vi "hse-application__GetSingleton.vi"(11 "Action":T1=enum."Get") -> (0 "Error Out":errorcluster, 3 "ApplicationClass DVR":refnum<data-value>)   [LabVIEW 2014, in "hse-application.lvclass"]
doc: "Contains the DVR to the HSE ApplicationClass object.\n\n____\nHAMPEL SOFTWARE ENGINEERING v0.12.0 (2018-09-13 18:21)"
uses:
  hse-application.lvclass
  hse-misc/Controls/FGV_Actions.ctl
  hse-misc/hse-misc.lvlib
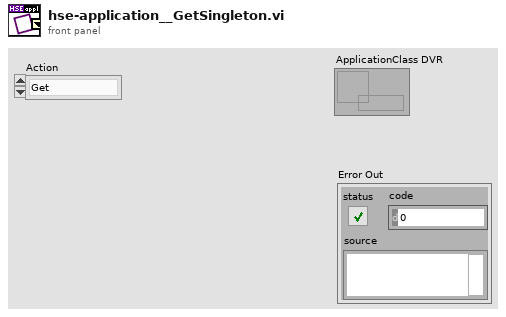
[diagram p1: front panel]
types:
  T1 = typedef "hse-misc.lvlib/FGV_Actions.ctl" = enum16{"Set", "Get"}
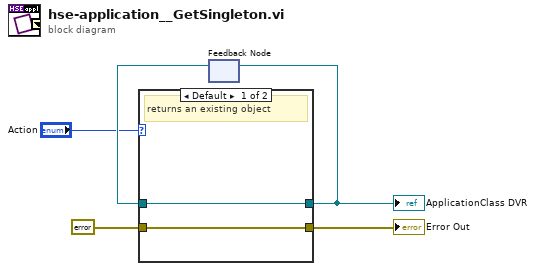
[diagram p0: block diagram]
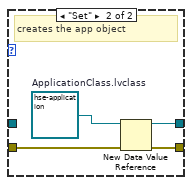
[diagram p2: hidden frame]
diagram:
  n1 = feedback #1() -> (w4:refnum<data-value>)  [unwired: 1 in]
  n2 = case shown="Default" "Action" {
    tunnel: [w7 w11] -> w5
    tunnel: w4 -> [w7 _]
    tunnel: [w6 w9] -> w2
    tunnel: errorcluster {"status"=FALSE, "code"=0, "source"=""} ("error out") -> [w6 w8]
    frame Default {
      # "returns an existing object"
    }
    frame "Set" {
      w10 = refnum<class "hse-application.lvclass"> refnum  # ApplicationClass.lvclass
      # "creates the app object"
      n3 = New Data Value Reference(data value=w10, error in=w8) -> (data value reference=w11:refnum<data-value>, error out=w9:errorcluster)
    }
  }
  "ApplicationClass DVR" <- w5
  "Error Out" <- w2
  n4 = feedback-in #1(w5) -> ()
